vi "To percent.vi"(8 "error in (no error)":errorcluster, 11 "I/p":dbl[](array[numeric])) -> (0 "error out":errorcluster, 3 "O/p":dbl[](array[numeric]))   [LabVIEW 2019, in "Zen Analytics.lvlib" / "Zen Analytics.lvclass"]
uses:
  Zen Analytics.lvclass
panel:
  # "array of values\na) Sum of all pass results\nb) Sum of all fail results"
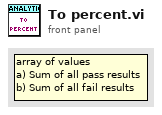
[diagram p1: front panel]
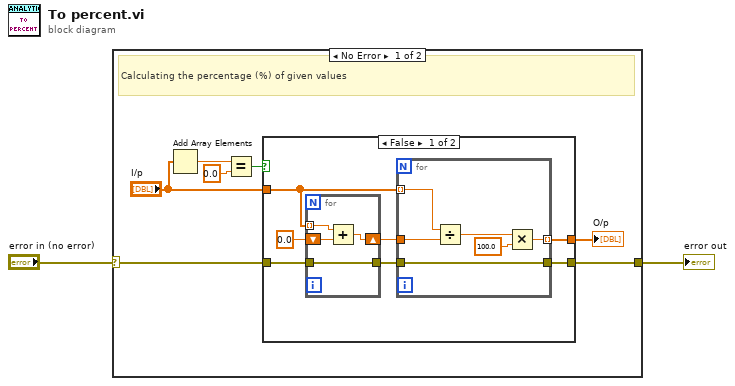
[diagram p0: block diagram]
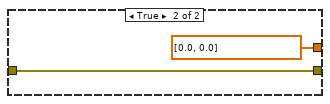
[diagram p2: hidden frame]
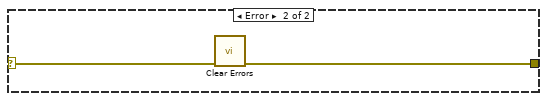
[diagram p3: hidden frame]
diagram:
  n1 = case shown="No Error" "error in (no error)" {
    selector: "error in (no error)" -> [w3 w30]
    tunnel: [w4 w29] -> w1
    frame No Error {
      # "Calculating the percentage (%) of given values"
      n2 = Add Array Elements(numeric array="I/p") -> (sum=w8:dbl)
      n3 = Equal?(x=w8, y=0.0 ("sum")) -> (x = y?=w5:bool)
      n4 = case shown="False" w5 {
        tunnel: "I/p" -> [w14 _]
        tunnel: [w13 dbl[] [0.0, 0.0]] -> w6
        tunnel: [w12 w27] -> w4
        tunnel: w3 -> [w10 w27]
        frame False {
          n5 = for {
            shift-right: [w26] -> w16
            shift-left: 0.0 -> [w25]
            tunnel: w14 -> [w24] mode=indexing
            tunnel: [w23] -> w11
            tunnel: w10 -> [w23]
            n6 = Add(x=w24, y=w25) -> (x+y=w26:dbl)
          }
          n7 = for {
            tunnel: w16 -> [w22]
            tunnel: w14 -> [w19] mode=indexing
            tunnel: [w18] -> w13 mode=indexing
            tunnel: [w17] -> w12
            tunnel: w11 -> [w17]
            n8 = Divide(x=w19, y=w22) -> (x/y=w21:dbl)
            n9 = Multiply(x=w21, y=100.0) -> (x*y=w18:dbl)
          }
        }
        frame True {
        }
      }
      "O/p" <- w6
    }
    frame Error {
      n10 = call <vilib>:"Clear Errors.vi"("error in (no error)"=w30) -> ("error out"=w29:errorcluster)  [unwired: 5 in, 1 out]
    }
  }
  "error out" <- w1
